vi "Unreserve Session.vi"(8 "error in":errorcluster, 10 "session information":T3, 11 "gRPC channel pool":T1) -> (0 "error out":errorcluster)   [LabVIEW 2020]
doc: "Unreserves the sessions based on the given session information."
uses:
  <vilib>/MeasurementLink/MeasurementLink Session Management Client/RPC Messages/ni_measurementlink_sessionmanagement_v1_SessionInformation.ctl
  <vilib>/MeasurementLink/MeasurementLink Session Management Client/RPC Messages/nidevice_grpc_Session.ctl
  <vilib>/MeasurementLink/MeasurementLink Session Management Client/RPC Messages/ni_measurementlink_sessionmanagement_v1_ChannelMapping.ctl
  GRPC Channel Pool.ctl
  <vilib>/gRPC/LabVIEW gRPC Library/Shared/grpcId.ctl
  <vilib>/MeasurementLink/MeasurementLink Session Management Client/MeasurementLink Session Management Client.lvlib
  <vilib>/gRPC/LabVIEW gRPC Library/grpc-lvsupport-release.lvlib
  NIDCPowerSourceDCVoltage.lvlib
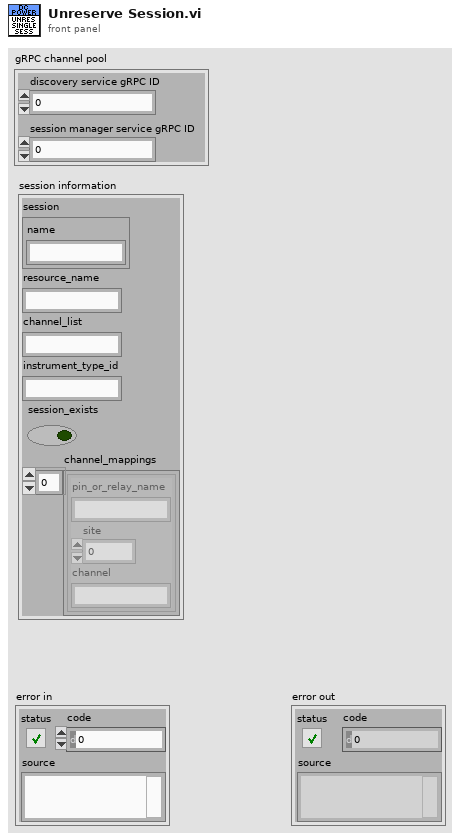
[diagram p1: front panel]
types:
  T1 = typedef "NIDCPowerSourceDCVoltage.lvlib/GRPC Channel Pool.ctl" = cluster{"discovery service gRPC ID":T2, "session manager service gRPC ID":T2}
  T2 = typedef "grpc-lvsupport-release.lvlib/grpcId.ctl" = u64
  T3 = typedef "MeasurementLink Session Management Client.lvlib/ni_measurementlink_sessionmanagement_v1_SessionInformation.ctl" = cluster{"session":T4, "resource_name":string, "channel_list":string, "instrument_type_id":string, "session_exists":bool, "channel_mappings":T5[]}
  T4 = typedef "MeasurementLink Session Management Client.lvlib/nidevice_grpc_Session.ctl" = cluster{"name":string}
  T5 = typedef "MeasurementLink Session Management Client.lvlib/ni_measurementlink_sessionmanagement_v1_ChannelMapping.ctl" = cluster{"pin_or_relay_name":string, "site":i32, "channel":string}
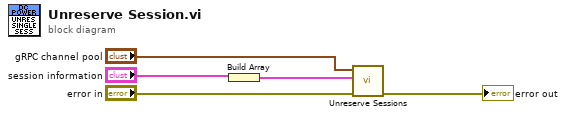
[diagram p0: block diagram]
diagram:
  n1 = Build Array("session information") -> (w1:T3[])
  n2 = call "Unreserve Sessions.vi"("error in"="error in", "session information"=w1, "gRPC channel pool"="gRPC channel pool") -> ("error out"=→"error out":errorcluster)  [unwired: 8 in]
